vi "HomeAutomation.vi"() -> ()   [LabVIEW 2020]
panel:
  in  "Speed":dbl(knob) scale=0.0..10.0
  in  "Stop":bool
  # "CLOUD"
  # "DATA RECIEVED"
  # "DATA SENT"
  # "SUBVI 1"
  # "SUBVI 2"
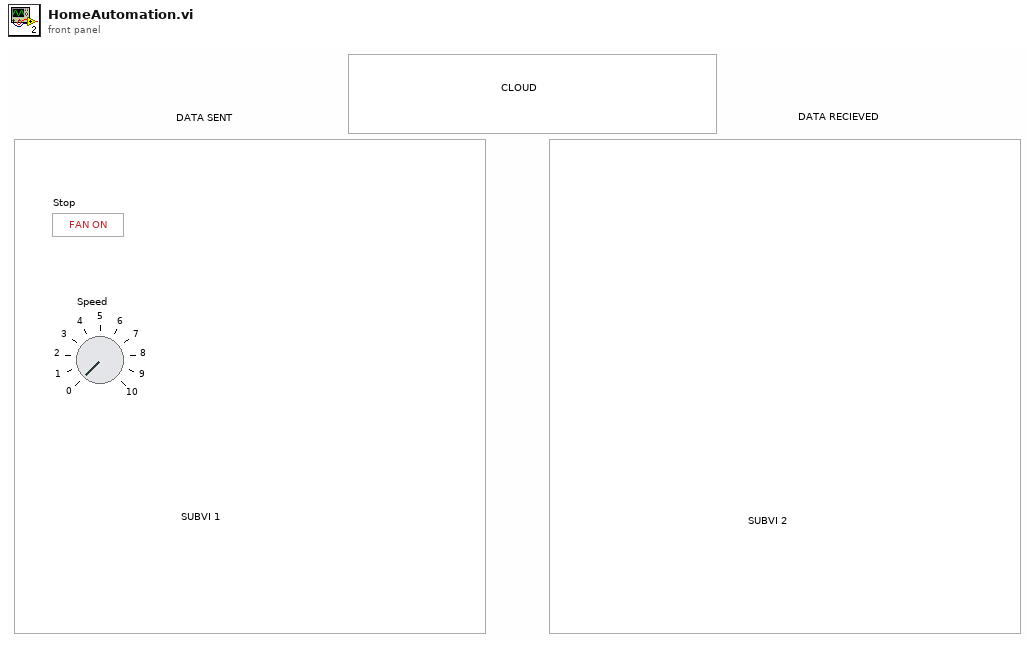
[diagram p1: front panel]
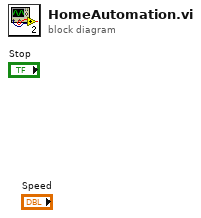
[diagram p0: block diagram]
diagram:
